vi "Fit N Gaussians.vi"(9 "Ellipse Data":cluster{"Major":dbl, "Minor":dbl}[](array[cluster]), 10 "Particle Reports (Pixels)":T3(array[cluster]), 11 "Image In":T1) -> (1 "Best-Fit Parameters":T2(array[cluster]), 2 "Best-Fit Image":T1, 3 "Image Src (Original)":T1)   [LabVIEW 2011]
uses:
  <vilib>/vision/Image Controls.llb/IMAQ Image.ctl
  <vilib>/gmath/NumericalOptimization/Nonlinear Curve Fit LM.vi
  <vilib>/gmath/NI_Gmath.lvlib
  <vilib>/vision/NI_Vision_Development_Module.lvlib
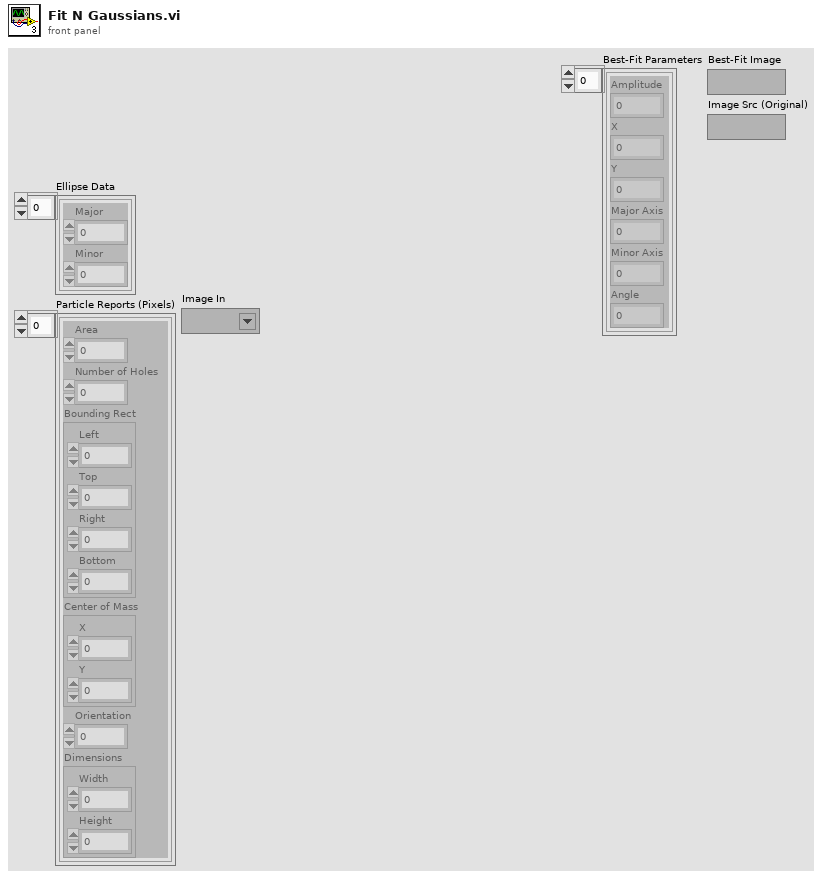
[diagram p1: front panel]
types:
  T1 = typedef "IMAQ Image.ctl" = refnum<image>
  T2 = cluster{"Amplitude":dbl, "X":dbl, "Y":dbl, "Major Axis":dbl, "Minor Axis":dbl, "Angle":dbl}[]
  T3 = cluster{"Area":dbl, "Number of Holes":dbl, "Bounding Rect":cluster{"Left":dbl, "Top":dbl, "Right":dbl, "Bottom":dbl}, "Center of Mass":cluster{"X":dbl, "Y":dbl}, "Orientation":dbl, "Dimensions":cluster{"Width":dbl, "Height":dbl}}[]
  T4 = typedef "Image Type" = u32
  T5 = cluster{"Width":i32, "Height":i32, "N Gaussians":i32}
  T6 = cluster{"Amplitude":dbl, "X":dbl, "Y":dbl, "Major Axis":dbl, "Minor Axis":dbl, "Angle":dbl}
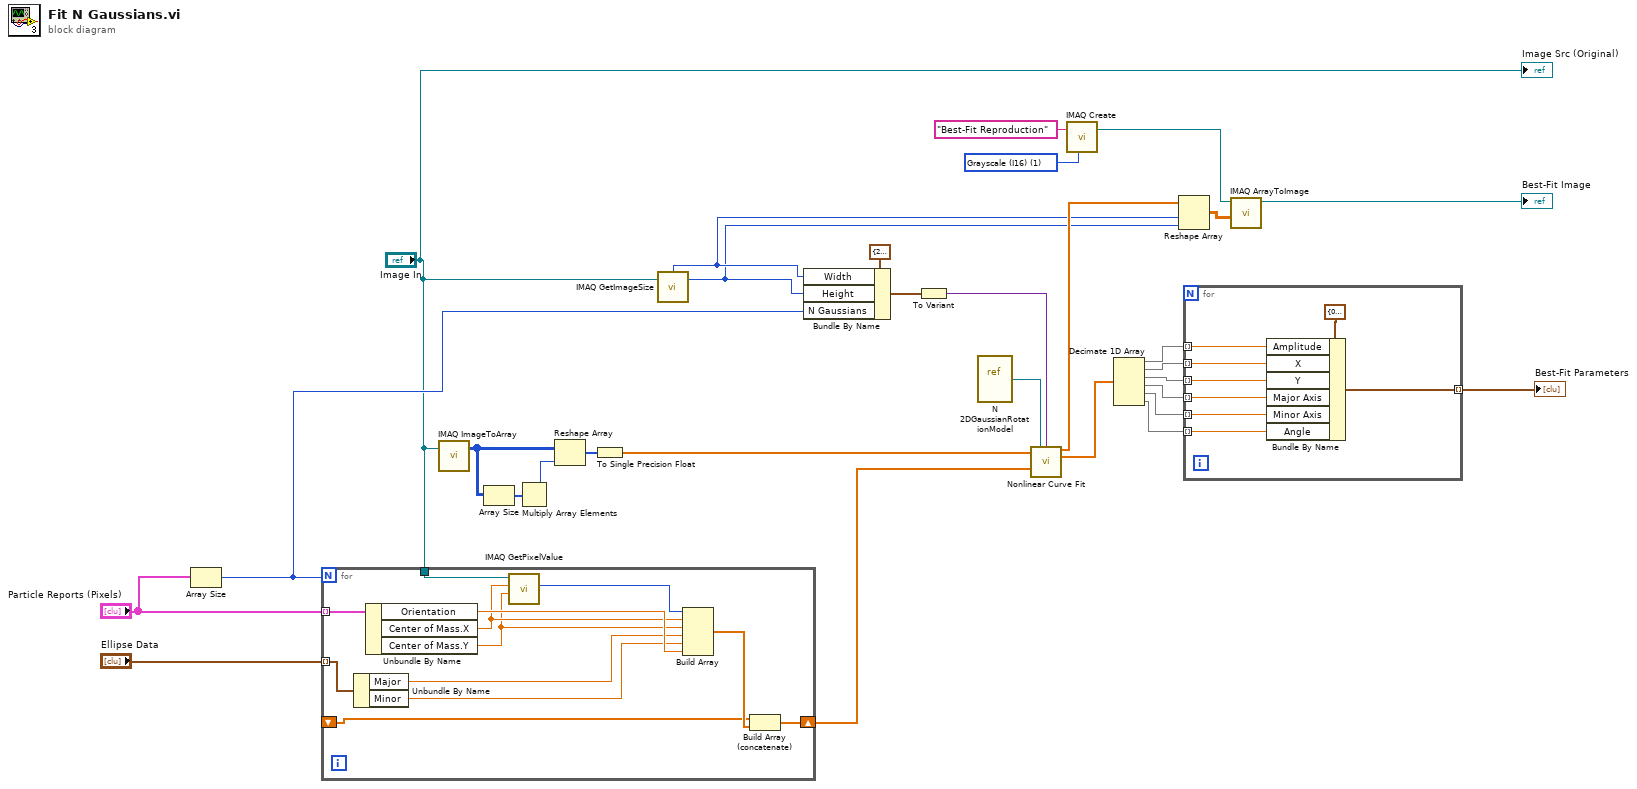
[diagram p0: block diagram]
diagram:
  w4 = T4 1 items=["Grayscale (U8)", "Grayscale (I16)", "Grayscale (SGL)", "Complex (CSG)", "RGB (U32)", "HSL (U32)", "RGB (U64)", "Grayscale (U16)"] ("Image Type")
  n1 = Array Size(array="Particle Reports (Pixels)") -> (size(s)=w18:i32)
  n2 = for {
    N: w18 -> [_]
    tunnel: "Particle Reports (Pixels)" -> [w42] mode=indexing
    tunnel: "Ellipse Data" -> [w36] mode=indexing
    tunnel: "Image In" -> [w37]
    shift-right: [w32] -> w19
    shift-left: _ -> [w31]
    n3 = Unbundle By Name(w36) -> ("Major"=w35:dbl, "Minor"=w34:dbl)
    n4 = Unbundle By Name(w42) -> ("Orientation"=w41:dbl, "Center of Mass.X"=w39:dbl, "Center of Mass.Y"=w38:dbl)
    n5 = call "IMAQ GetPixelValue"("Image"=w37, "X Coordinate"=w39, "Y Coordinate"=w38) -> ("Pixel Value (I16)"=w40:i16)  [unwired: 3 in, 4 out]
    n6 = Build Array(w40, w39, w38, w35, w34, w41) -> (w33:dbl[])
    n7 = Build Array (concatenate)(w31, w33) -> (w32:dbl[])
  }
  n8 = call "IMAQ ImageToArray"("Image"="Image In") -> ("Image Pixels (I16)"=w24:i16[][])  [unwired: 3 in, 4 out]
  n9 = Array Size(array=w24) -> (size(s)=w25:i32[])
  n10 = Multiply Array Elements(1:w25) -> (0:w26:i32)
  n11 = Reshape Array(w24, w26) -> (w23:i16[])
  n12 = To Single Precision Float(number=w23) -> (single precision float=w22:sgl[])
  n13 = call "IMAQ GetImageSize"("Image"="Image In") -> ("Y Resolution"=w7:i32, "X Resolution"=w8:i32)  [unwired: 3 in, 1 out]
  n14 = Bundle By Name(cluster=T5 {"Width"=25, "Height"=25, "N Gaussians"=2}, "Width"=w8, "Height"=w7, "N Gaussians"=w18) -> (w29:T5)
  n15 = To Variant(anything=w29) -> (Variant=w27:variant)
  n16 = vi-ref "N 2DGaussianRotationModel.vi"() -> (w30:refnum<vi>)
  n17 = call-poly <vilib>:"Nonlinear Curve Fit.vi"("Y"=w22, "f(x,a)"=w30, "data"=w27, "initial parameters"=w19) -> ("best nonlinear fit"=w9:dbl[], "best fit parameters"=w17:dbl[])  [unwired: 6 in, 4 out]
  n18 = call "IMAQ Create"("Image Name"="Best-Fit Reproduction", "Image Type"=w4) -> ("New Image"=w3:T1)  [unwired: 3 in, 1 out]
  n19 = Decimate 1D Array(w17) -> (w16:dbl[], w15:dbl[], w14:dbl[], w13:dbl[], w12:dbl[], w11:dbl[])
  n20 = Reshape Array(w9, w8, w7) -> (w6:dbl[][])
  n21 = for {
    tunnel: w16 -> [w49] mode=indexing
    tunnel: w15 -> [w48] mode=indexing
    tunnel: w14 -> [w47] mode=indexing
    tunnel: w13 -> [w46] mode=indexing
    tunnel: w12 -> [w45] mode=indexing
    tunnel: w11 -> [w44] mode=indexing
    tunnel: [w43] -> w10 mode=indexing
    n22 = Bundle By Name(cluster=T6 {"Amplitude"=0.0, "X"=0.0, "Y"=0.0, "Major Axis"=0.0, "Minor Axis"=0.0, "Angle"=0.0}, "Amplitude"=w49, "X"=w48, "Y"=w47, "Major Axis"=w46, "Minor Axis"=w45, "Angle"=w44) -> (w43:T6)
  }
  "Best-Fit Parameters" <- w10
  n23 = call "IMAQ ArrayToImage"("Image Pixels (I16)"=w6, "Image"=w3) -> ("Image Out"=→"Best-Fit Image":T1)  [unwired: 8 in, 1 out]
  "Image Src (Original)" <- "Image In"
